vi "Smart Factory Demo.vi"() -> ()   [LabVIEW 2015]
uses:
  <vilib>/Utility/tdmsutil.llb/fileViewerConfigData.ctl
  <vilib>/addons/_XControls/Orbit Plot/SVX Orbit.xctl
  <vilib>/LabSocket/LabSocket.lvlib
panel:
  in  "stop":bool
  out "url":string
  out "LastXScaleFormat":u8
  out "TotalCount":u64
  out "Temp Configuration":T1
  in  "LastTopLeftValue":u64
  out "Resize?":bool
  in  "Help":bool
  out "file path out":path
  in  "Status":string
  in  "Quit":bool
  in  "Settings...":bool
  out "error out":errorcluster
  in  "error in (no error)":errorcluster
  in  "file path":path
  in  "Boolean Text.Text":string
  in  "Color Box 2":u32(colorbox)
  in  "Color Box":u32(colorbox)
  in  "Change Color":bool
  in  "Tab Control":T2(tab)
  out "Boolean 3":bool
  out "Boolean 5":bool
  out "Boolean 2":bool
  out "Waveform Chart 2":dbl(graph)
  out "Waveform Chart":dbl(graph)
  out "Waveform Graph":waveform(dbl)[](graph)
  in  "File contents":string(tree)
  out "Orbit Plot":T3(xcontrol)
  out "Full Spectrum":T4(graph)
  out "Voltage Harmonic Spectra":T5(graph)
  in  "Raw Data":string[][](table)=[["3", "4", "1", "6", "2"], ["33", "26", "12", "100", "23"], ["4", "3", "1", "8", "2"], ["4", "8", "4", "12", "4"], ["2", "3", "1", "9", "3"], ["3", "2", "3", "12", "1"]]
  out "Stacked Bar Plots":dbl[][](graph)
  in  "Stop":bool
  in  "OK Button 3":bool
  in  "OK Button 2":bool
  in  "OK Button":bool
  # "Smart Factory Demonstration"
  # "Dashboard"
  # "123 (2)"
  # "123 (2)"
  # "16%"
  # "37 C"
  # "Warning"
  # "Alarm"
  # "Used storage"
  # "Equipment Overview"
  # "Overview: Illustrates the use of the waveform graph to display stacked bar plots.\nInstructions:\nRun the VI."
  # "Stacked Bar Waveform Graph.vi"
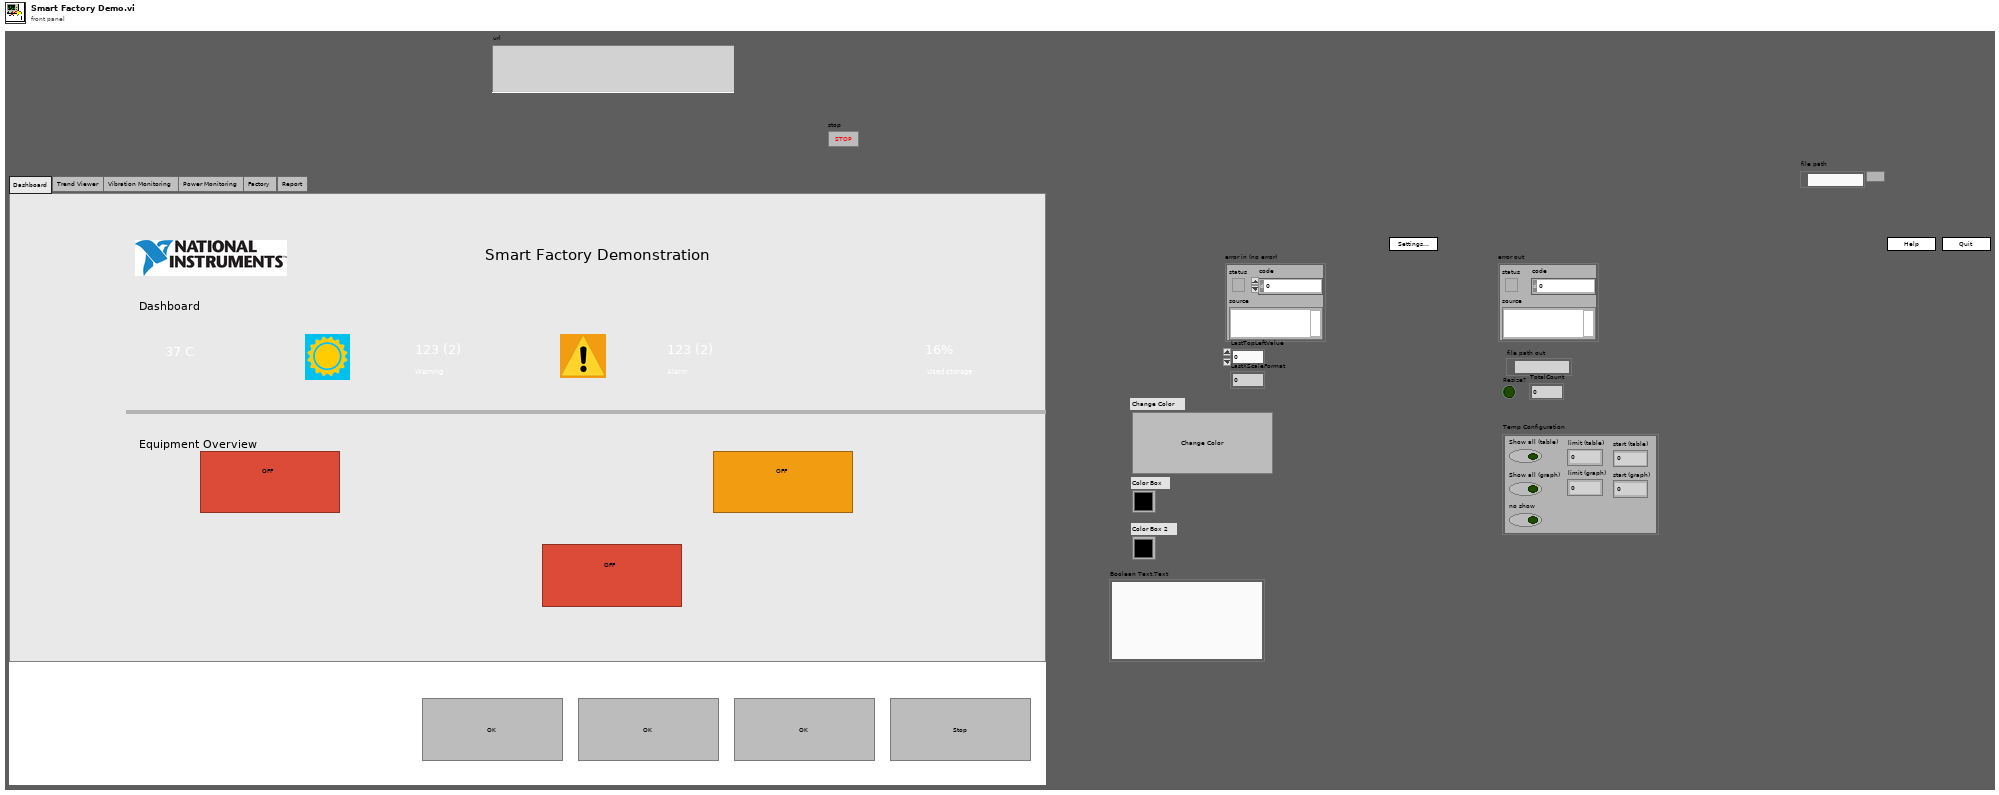
[diagram p1: front panel]
types:
  T1 = typedef "fileViewerConfigData.ctl" = cluster{"Show all (table)":bool, "Show all (graph)":bool, "limit (table)":u64, "limit (graph)":u64, "no show":bool, "start (table)":u64, "start (graph)":u64}
  T2 = enum32{"Dashboard", "Trend Viewer", "Vibration Monitoring", "Power Monitoring", "Factory", "Report"}
  T3 = cluster{"probe x":dbl[], "probe y":dbl[], "reference":dbl[], "plot type":enum16{"Filtered Plot", "Unfiltered Plot"}, "attribute":variant}[][]
  T4 = cluster{"Order 0":dbl, "dOrder":dbl, "magnitude":dbl[]}[]
  T5 = cluster{"order 0":dbl, "delta order":dbl, "complex spectrum":dbl[]}[]
  T6 = cluster{"LabSocket_Server":string, "External":string}
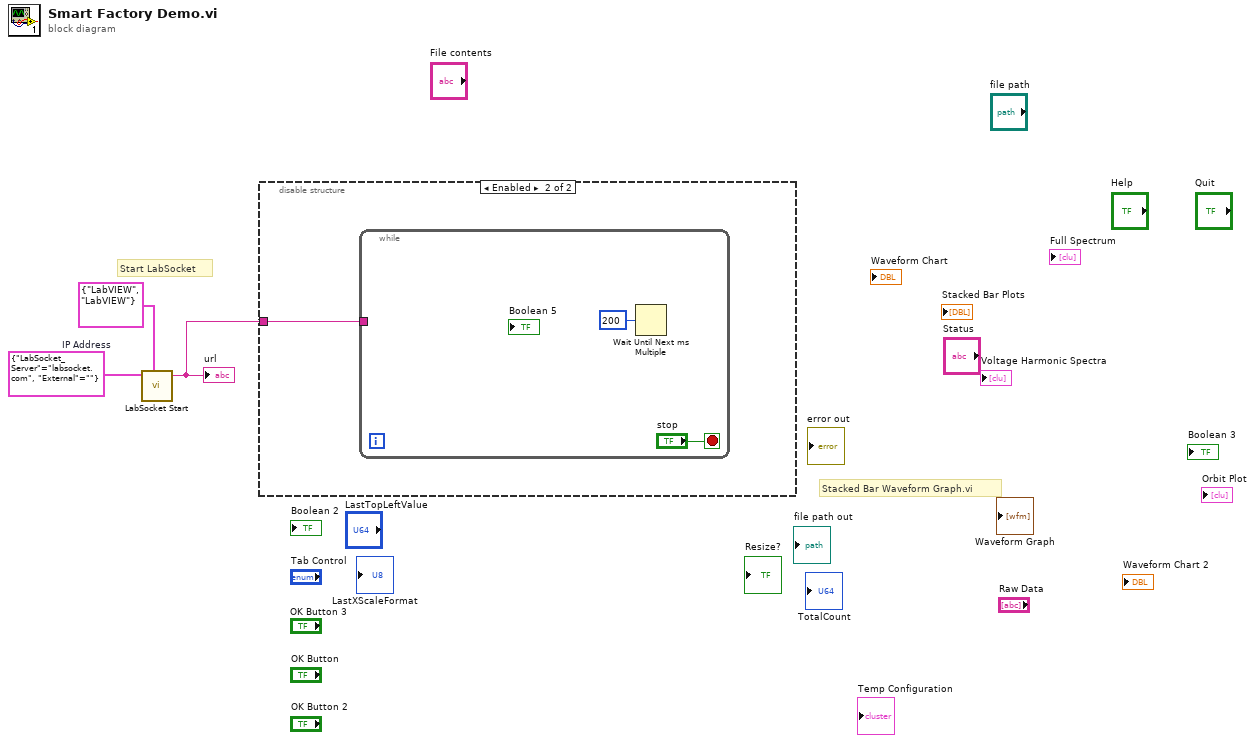
[diagram p0: block diagram]
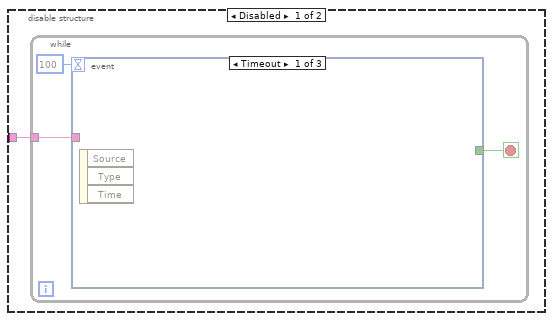
[diagram p2: hidden frame]
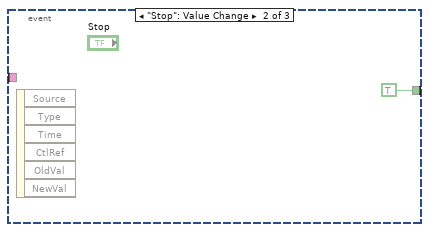
[diagram p3: hidden frame]
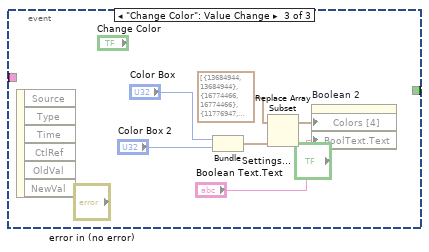
[diagram p4: hidden frame]
diagram:
  w3 = T6 {"LabSocket_Server"="labsocket.com", "External"=""}  # IP Address
  # "Start LabSocket"
  # "Stacked Bar Waveform Graph.vi"
  n1 = call <vilib>:"LabSocket Start.vi"("Server Credentials \n(LabVIEW/LabVIEW)"=cluster{"User Name":string, "Password":string} {"User Name"="LabVIEW", "Password"="LabVIEW"} ("Server Credentials \n(guest/guest)"), "IP Address"=w3) -> ("URL"=w1:string)  [unwired: 8 in, 1 out]
  "url" <- w1
  n2 = disable-structure shown="Enabled" {
    disable-tunnel: w1 -> [w4 w15]
    frame Disabled {
      n3 = while {
        tunnel: w4 -> [w5]
        stop <- w7 stop-if-true
        n4 = event shown="[0] Timeout" {
          selector: _ -> [_ _ _]
          dyn-events: _ -> [_ _ _]
          timeout: 100 -> [_ _ _]
          tunnel: [_ TRUE _] -> w7
          tunnel: w5 -> [_ _ _]
          event Timeout {
            n5 = event-data() -> ()  [unwired: 1 in, 3 out]
          }
          event "Stop": Value Change {
            n6 = event-data() -> ()  [unwired: 1 in, 6 out]
          }
          event "Change Color": Value Change {
            n7 = event-data() -> ()  [unwired: 1 in, 6 out]
            n8 = Bundle("Color Box"="Color Box", "Color Box 2"="Color Box 2") -> (w11:cluster{"Color Box":u32, "Color Box 2":u32})  [unwired: 1 in]
            n9 = Replace Array Subset(array=cluster{u32, u32}[] [{13684944, 13684944}, {16774466, 16774466}, {11776947, 39168}, {11776947, 39168}] ("Colors [4]"), new element=w11) -> (w10:cluster{u32, u32}[])  [unwired: 1 in]
            n10 = property on="Boolean 2" class="Bool (strict)"("Colors [4]"=w10, "BoolText.Text"="Boolean Text.Text") -> ()  [unwired: 2 in, 2 out]
          }
        }
      }
    }
    frame Enabled {
      n11 = while {
        tunnel: w15 -> [_]
        stop <- "stop" stop-if-true
        n12 = Wait Until Next ms Multiple(millisecond multiple=u32 200) -> ()  [unwired: 1 out]
      }
    }
  }
